vi "Get_Profile_pathess.vi"(8 "error in (no error)":errorcluster, 10 "Target?":bool, 11 "OSArch":string) -> (0 "error out":errorcluster, 3 "profileDestPath":string)   [LabVIEW 2016, in "Scan Engine Custom Device.lvlib"]
uses:
  Scan Engine Custom Device.lvlib
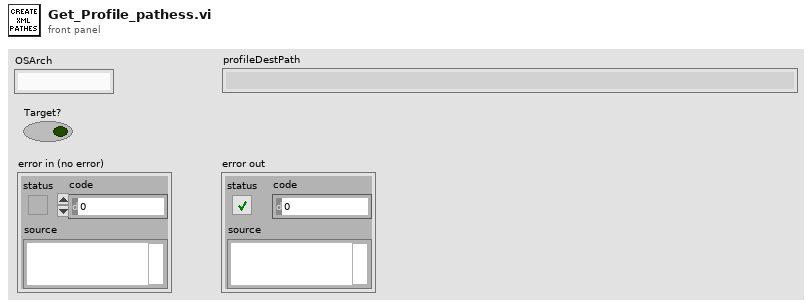
[diagram p1: front panel]
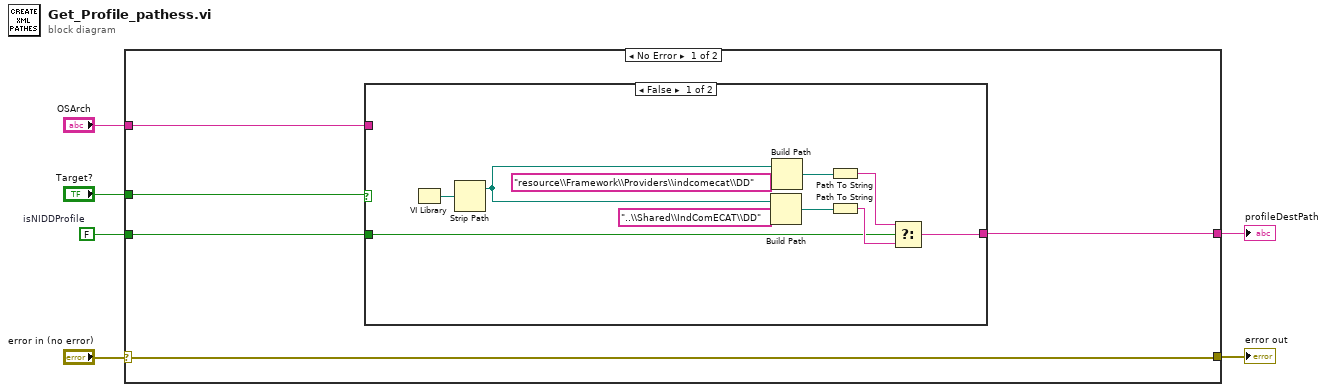
[diagram p0: block diagram]
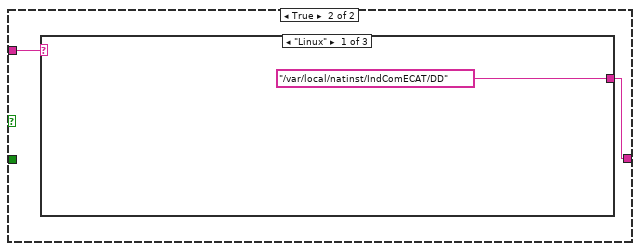
[diagram p2: hidden frame]
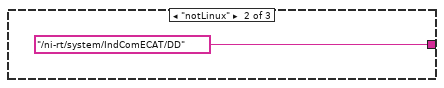
[diagram p3: hidden frame]
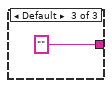
[diagram p4: hidden frame]
diagram:
  w1 = FALSE  # isNIDDProfile
  n1 = case shown="No Error" "error in (no error)" {
    selector: "error in (no error)" -> [w11 w27]
    tunnel: "OSArch" -> [w10 _]
    tunnel: [w11 w27] -> w5
    tunnel: "Target?" -> [w9 _]
    tunnel: [w8 _] -> w2
    tunnel: w1 -> [w7 _]
    frame No Error {
      n2 = case shown="False" w9 {
        tunnel: w7 -> [w12 _]
        tunnel: w10 -> [_ w23]
        tunnel: [w13 w22] -> w8
        frame False {
          n3 = VI Library() -> (path=w16:path)
          n4 = Strip Path(path=w16) -> (stripped path=w19:path)  [unwired: 1 out]
          n5 = Build Path(base path=w19, name or relative path="..\\Shared\\IndComECAT\\DD") -> (appended path=w18:path)
          n6 = Build Path(base path=w19, name or relative path="resource\\Framework\\Providers\\indcomecat\\DD") -> (appended path=w21:path)
          n7 = Path To String(path=w21) -> (string=w15:string)
          n8 = Path To String(path=w18) -> (string=w14:string)
          n9 = Select(t=w15, s=w12, f=w14) -> (s? t:f=w13:string)
        }
        frame True {
          n10 = case shown="\"Linux\"" w23 {
            tunnel: ["/var/local/natinst/IndComECAT/DD" "/ni-rt/system/IndComECAT/DD" ""] -> w22
            frame "Linux" {
            }
            frame "notLinux" {
            }
            frame Default {
            }
          }
        }
      }
    }
    frame Error {
    }
  }
  "error out" <- w5
  "profileDestPath" <- w2
